vi "SpreadsheetReadExpress.vi"() -> ()   [LabVIEW 2015]
panel:
  out "XY Graph":cluster{"all rows":dbl[], "all rows":dbl[]}(graph)
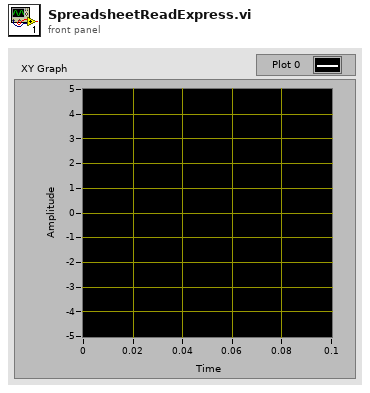
[diagram p1: front panel]
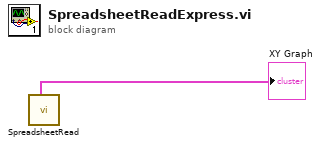
[diagram p0: block diagram]
diagram:
  n1 = call "SpreadsheetRead.vi"() -> ("XY Graph"=→"XY Graph":cluster{"all rows":dbl[], "all rows":dbl[]})  [unwired: 11 in]
